vi "Load Plugins.vi"(8 "error in (no error)":errorcluster, 11 "Plugin Directories":path[](array[path])) -> (0 "error out":errorcluster, 3 "Plugin Array":T1[](array[typedef]))   [LabVIEW 2020, in "Plugin Manager.lvlib"]
uses:
  Plugin Manager.lvlib
  Plugin Details.ctl
  Plugin Servers/Controller/Controller Type.ctl
  Plugin Types.ctl
  Plugin Servers/Controller/Generic Plugin.lvclass
panel:
  out "All Files in Dir":path[](array[path])
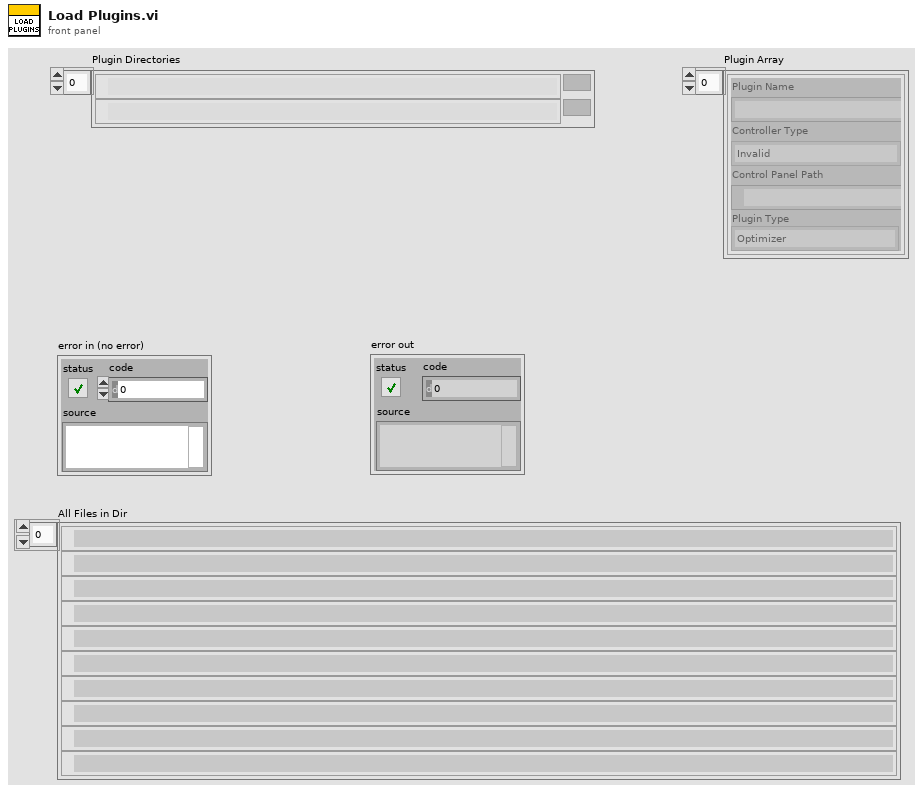
[diagram p1: front panel]
types:
  T1 = typedef "Plugin Manager.lvlib/Plugin Details.ctl" = cluster{"Plugin Name":string, "Controller Type":T2, "Control Panel Path":path, "Plugin Type":T3}
  T2 = typedef "Generic Plugin.lvclass/Controller Type.ctl" = enum16{"Invalid", "Temperature Controller", "Pump Controller", "Generic Optimizer", "LC Parser"}
  T3 = typedef "Plugin Manager.lvlib/Plugin Types.ctl" = enum16{"Invalid", "Optimizer", "Analyzer", "Hardware"}
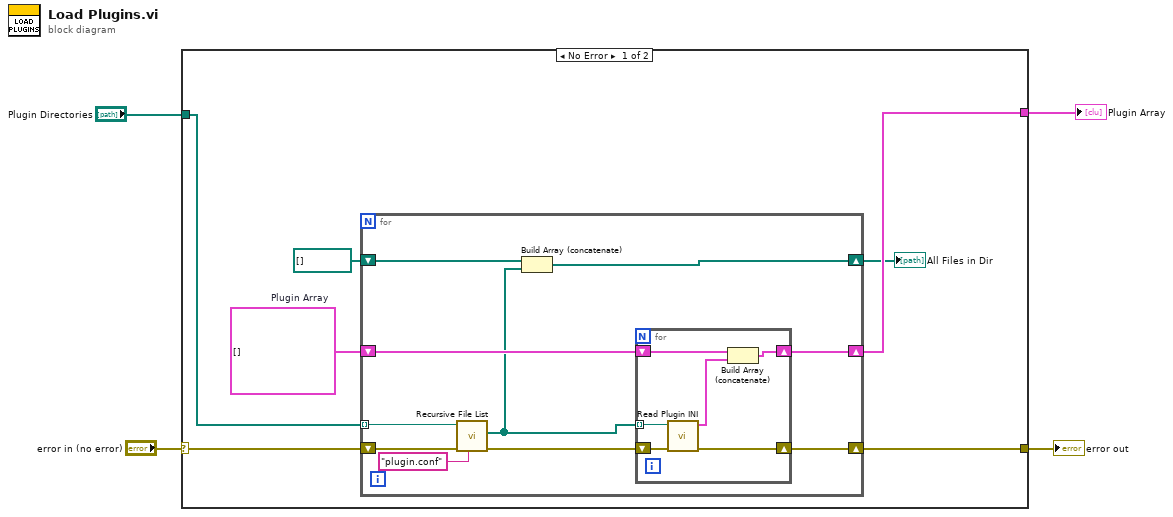
[diagram p0: block diagram]
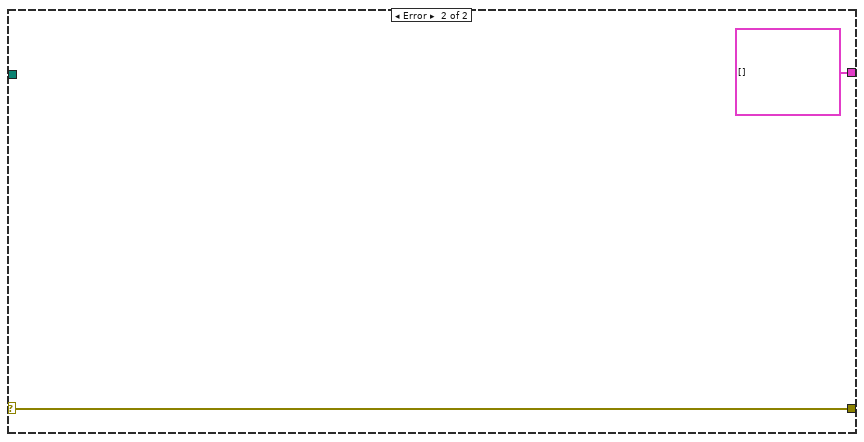
[diagram p2: hidden frame]
diagram:
  n1 = case shown="No Error" "error in (no error)" {
    selector: "error in (no error)" -> [w11 w29]
    tunnel: [w10 w29] -> w3
    tunnel: "Plugin Directories" -> [w7 _]
    tunnel: [w8 T1[] [] ("Plugin Array")] -> w2
    frame No Error {
      w9 = T1[] []  # Plugin Array
      n2 = for {
        shift-right: [w18] -> w10
        shift-left: w11 -> [w21]
        shift-right: [w16] -> w8
        shift-left: w9 -> [w17]
        tunnel: w7 -> [w15] mode=indexing
        shift-right: [w13] -> w6
        shift-left: path[] [] ("All Files in Dir") -> [w14]
        n3 = call <vilib>:"Recursive File List.vi"("pattern"="plugin.conf", "error in (no error)"=w21, "Folder Path"=w15) -> ("error out"=w19:errorcluster, "All Files in Dir"=w12:path[])  [unwired: 4 in, 3 out]
        n4 = Build Array (concatenate)(w14, w12) -> (w13:path[])
        n5 = for {
          shift-right: [w26] -> w18
          shift-left: w19 -> [w27]
          tunnel: w12 -> [w25] mode=indexing
          shift-right: [w23] -> w16
          shift-left: w17 -> [w24]
          n6 = call "Read Plugin INI.vi"("error in (no error)"=w27, "INI file"=w25) -> ("error out"=w26:errorcluster, "Plugin Details"=w22:T1)  [unwired: 8 in]
          n7 = Build Array (concatenate)(w24, w22) -> (w23:T1[])
        }
      }
      "All Files in Dir" <- w6
    }
    frame Error {
    }
  }
  "error out" <- w3
  "Plugin Array" <- w2
